vi "is slow response a fire command.vi"(11 "Expected slow response":string) -> (3 "False is Fire cmd":bool)   [LabVIEW 2018]
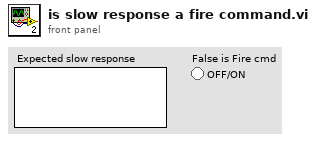
[diagram p1: front panel]
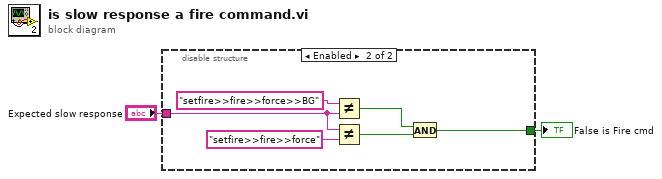
[diagram p0: block diagram]
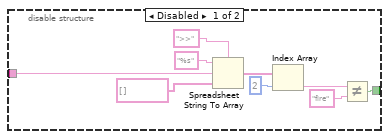
[diagram p2: hidden frame]
diagram:
  n1 = disable-structure shown="Enabled" {
    disable-tunnel: "Expected slow response" -> [w11 w15]
    disable-tunnel: [w10 w12] -> w1
    frame Disabled {
      n2 = Spreadsheet String To Array(delimiter (Tab)=">>", format string="%s", spreadsheet string=w11, array type (2D Dbl)=string[] []) -> (array=w7:string[])
      n3 = Index Array(array=w7, index=2) -> (element=w9:string)
      n4 = Not Equal?(x=w9, y="fire") -> (x != y?=w10:bool)
    }
    frame Enabled {
      n5 = Not Equal?(x="setfire>>fire>>force>>BG" ("Command to Send"), y=w15) -> (x != y?=w14:bool)
      n6 = Not Equal?(x=w15, y="setfire>>fire>>force") -> (x != y?=w13:bool)
      n7 = And(x=w14, y=w13) -> (x .and. y?=w12:bool)
    }
  }
  "False is Fire cmd" <- w1
